vi "Get Control Value.vi"(7 "Control Reference":refnum<vi>, 8 "error in (no error)":errorcluster, 9 "Control Index":i32, 10 "No Control Index":bool, 11 "VI Reference":refnum<vi>) -> (0 "error out":errorcluster, 3 "Variant":variant)   [LabVIEW 2017, in "Front Panel Publisher.lvlib" / "Control.lvclass"]
uses:
  Control.lvclass
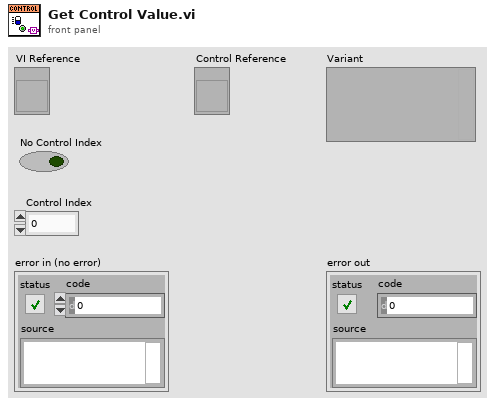
[diagram p1: front panel]
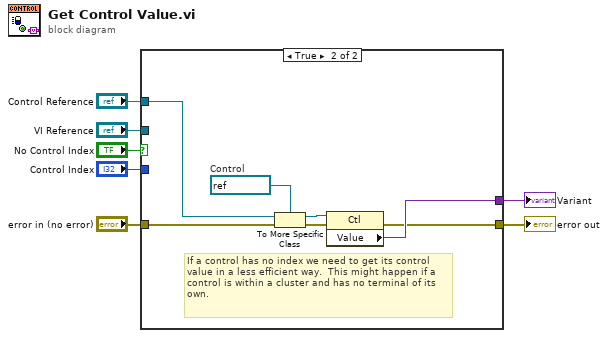
[diagram p0: block diagram]
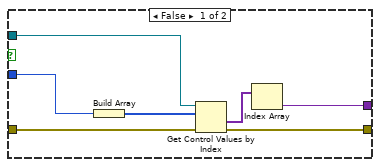
[diagram p2: hidden frame]
diagram:
  n1 = case shown="True" "No Control Index" {
    tunnel: "VI Reference" -> [w14 _]
    tunnel: "error in (no error)" -> [w13 w19]
    tunnel: [w12 w16] -> w5
    tunnel: [w11 w15] -> w4
    tunnel: "Control Index" -> [w10 _]
    tunnel: "Control Reference" -> [_ w21]
    frame False {
      n2 = Build Array(w10) -> (w9:i32[])
      n3 = Get Control Values by Index(0:w14, 1:w9, 3:w13) -> (10:w8:variant[], 11:w11:errorcluster)
      n4 = Index Array(array=w8) -> (element=w12:variant)  [unwired: 1 in]
    }
    frame True {
      w17 = refnum<vi> refnum  # Control
      # "If a control has no index we need to get its control value in a less efficient way.  This might happen if a control is within a cluster and has no terminal of its own."
      n5 = To More Specific Class(target class=w17, reference=w21, error in=w19) -> (specific class reference=w20:refnum<vi>, error out=w18:errorcluster)
      n6 = property class="Ctl"(reference=w20, error in=w18) -> (error out=w15:errorcluster, "Value"=w16:variant)  [unwired: 1 out]
    }
  }
  "Variant" <- w5
  "error out" <- w4
